vi "Write Pin.vi"(0 "Cypress in":refnum<class "Cypress.lvclass">, 5 "VISA resource name":refnum<visa-resource-name>, 7 "Pin":u16, 9 "Port 3":u16, 11 "error in (no error)":errorcluster, 12 "Set Pin":bool) -> (4 "Cypress out":refnum<class "Cypress.lvclass">, 6 "VISA resource name 2":refnum<visa-resource-name>, 15 "error out":errorcluster)   [LabVIEW 2020, in "Cypress.lvclass"]
uses:
  Cypress.lvclass
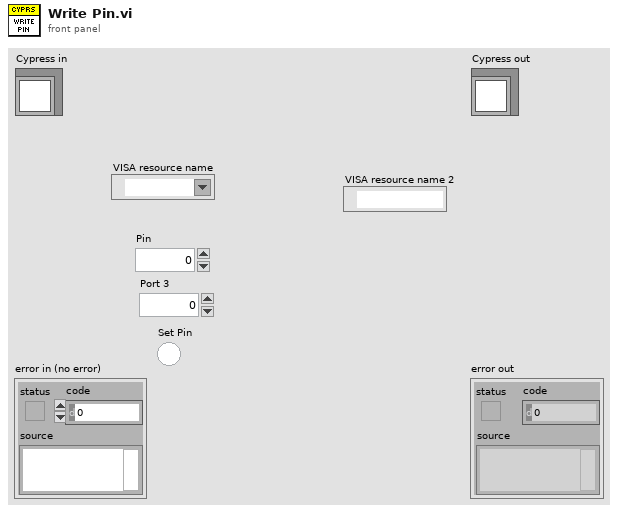
[diagram p1: front panel]
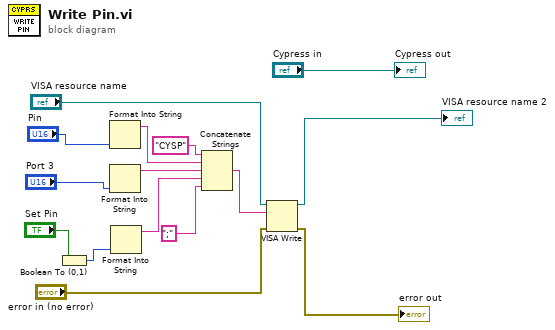
[diagram p0: block diagram]
diagram:
  n1 = Boolean To (0,1)(Boolean="Set Pin") -> (0, 1=w1:i16)
  n2 = Format Into String("Pin") -> (resulting string=w13:string)  [unwired: 3 in, 1 out]
  n3 = Format Into String("Port 3") -> (resulting string=w12:string)  [unwired: 3 in, 1 out]
  n4 = Format Into String(w1) -> (resulting string=w9:string)  [unwired: 3 in, 1 out]
  n5 = Concatenate Strings("CYSP" ("string"), w13, w12, w9, ";" ("string")) -> (w3:string)
  n6 = VISA Write(VISA resource name="VISA resource name", write buffer=w3, error in (no error)="error in (no error)") -> (VISA resource name out=→"VISA resource name 2":refnum<visa-resource-name>, error out=→"error out":errorcluster)  [unwired: 1 out]
  "Cypress out" <- "Cypress in"
